vi "downramp.vi"(11 "number of steps":i32=50) -> (3 "downramp array":dbl[](array[numeric]))   [LabVIEW 2020]
panel:
  out "downramp array 3":dbl[](graph)
  out "downramp array 2":dbl[](graph)
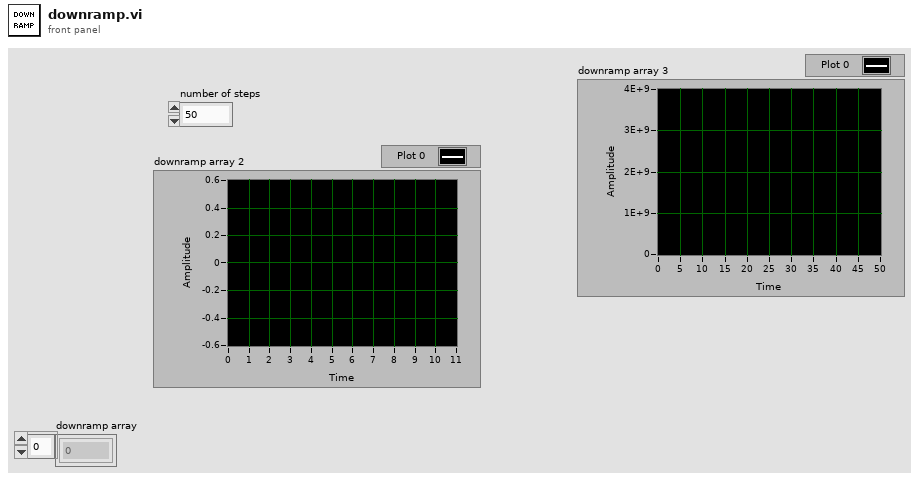
[diagram p1: front panel]
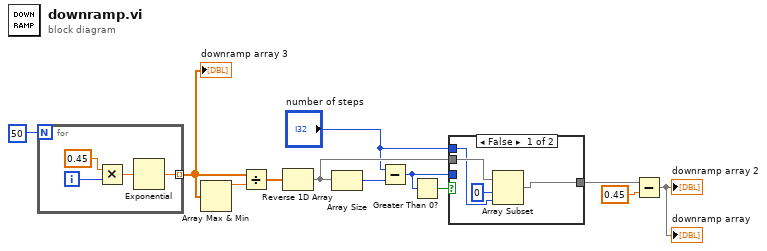
[diagram p0: block diagram]
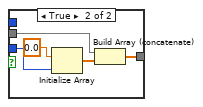
[diagram p2: hidden frame]
diagram:
  n1 = for {
    N: 50 -> [_]
    tunnel: [w16] -> w10 mode=indexing
    i -> [w15]
    n2 = Multiply(x=0.45, y=w15) -> (x*y=w13:dbl)
    n3 = Exponential(1:w13) -> (0:w16:dbl)
  }
  "downramp array 3" <- w10
  n4 = Array Max & Min(array=w10) -> (max value=w12:dbl)  [unwired: 3 out]
  n5 = Divide(x=w10, y=w12) -> (x/y=w9:dbl[])
  n6 = Reverse 1D Array(array=w9) -> (reversed array=w6:dbl[])
  n7 = Array Size(array=w6) -> (size(s)=w4:i32)
  n8 = Subtract(x="number of steps", y=w4) -> (x-y=w3:i32)
  n9 = Greater Than 0?(x=w3) -> (x > 0?=w2:bool)
  n10 = case shown="False" w2 {
    tunnel: w6 -> [w20 w25]
    tunnel: [w18 w24] -> w5
    tunnel: w3 -> [_ w23]
    tunnel: "number of steps" -> [w17 _]
    frame False {
      n11 = Array Subset(array=w20, index=0, length=w17) -> (w18:dbl[])
    }
    frame True {
      n12 = Initialize Array(0.0 ("element"), w23) -> (w21:dbl[])
      n13 = Build Array (concatenate)(w25, w21) -> (w24:dbl[])
    }
  }
  n14 = Subtract(x=w5, y=0.45 ("x")) -> (x-y=→"downramp array" →"downramp array 2":dbl[])
